vi "Open_ESP.vi"(8 "error in (no error)":errorcluster, 9 "Baudrate":i64, 11 "Selector":string(combo)) -> (0 "error out":errorcluster, 2 "find list":string[](array[string]), 3 "VISA resource name out":refnum<visa-resource-name>)   [LabVIEW 2025]
uses:
  <vilib>/Instr/_visa.llb/VISA Configure Serial Port (Instr).vi
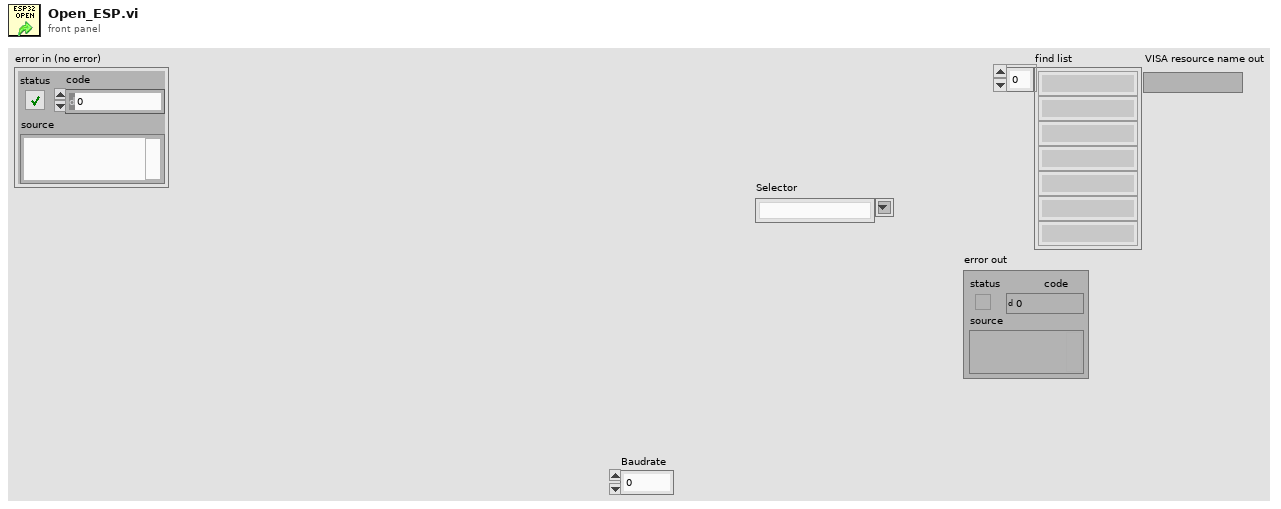
[diagram p1: front panel]
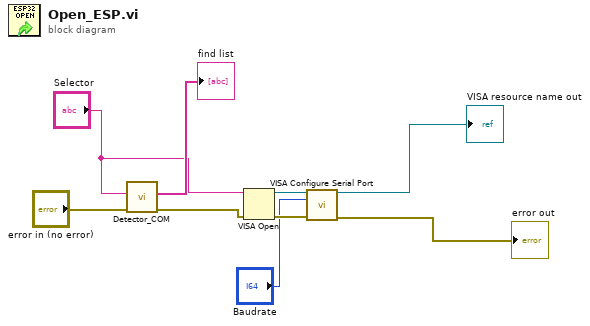
[diagram p0: block diagram]
diagram:
  n1 = call "Detector_COM.vi"("error in (no error)"="error in (no error)", "Selector"="Selector") -> ("error out"=w6:errorcluster, "find list"=→"find list":string[])  [unwired: 8 in]
  n2 = VISA Open(error in (no error)=w6, VISA resource name="Selector") -> (VISA resource name=w9:refnum<visa-resource-name>, error out=w5:errorcluster)  [unwired: 3 in]
  n3 = call-poly "VISA Configure Serial Port"("VISA resource name"=w9, "baud rate (9600)"="Baudrate", "error in (no error)"=w5) -> ("VISA resource name out"=→"VISA resource name out":refnum<visa-resource-name>, "error out"=→"error out":errorcluster)  [unwired: 11 in]
